vi "Card.vi"(7 "Mode":T1(ring), 8 "error in (no error)":errorcluster, 10 "Queue In":cluster{"Certificate":bool, "Card Info":string}={"Certificate"=TRUE, "Card Info"=""}) -> (0 "error out":errorcluster, 2 "Queue Out":cluster{"Certificate":bool, "Card Info":string}={"Certificate"=TRUE, "Card Info"=""})   [LabVIEW 2011]
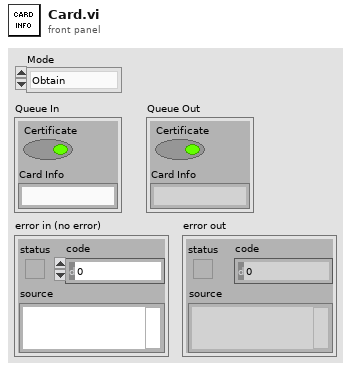
[diagram p1: front panel]
types:
  T1 = enum16{"Obtain", "Enqueue", "Dequeue", "Release"}
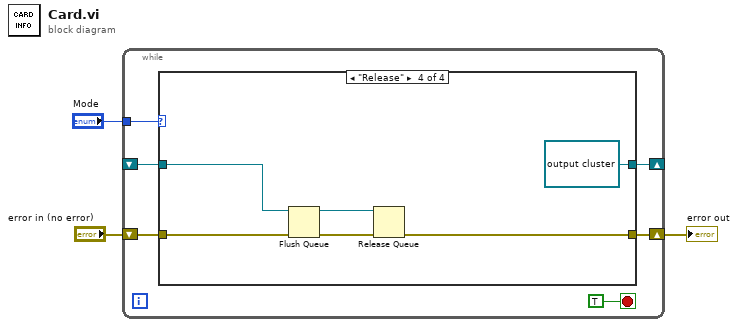
[diagram p0: block diagram]
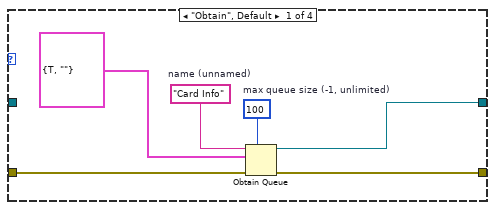
[diagram p2: hidden frame]
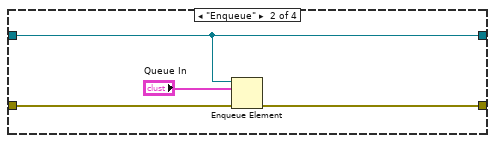
[diagram p3: hidden frame]
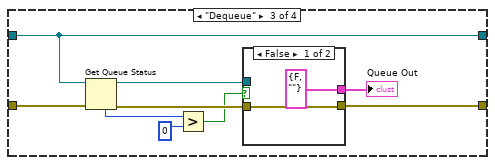
[diagram p4: hidden frame]
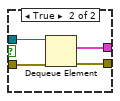
[diagram p5: hidden frame]
diagram:
  n1 = while {
    tunnel: "Mode" -> [w9]
    shift-right: [w7] -> w1
    shift-left: "error in (no error)" -> [w8]
    shift-right: [w6] -> _
    shift-left: _ -> [w5]
    stop <- TRUE stop-if-true
    n2 = case shown="\"Release\"" w9 {
      tunnel: w8 -> [w15 w19 w27 w36]
      tunnel: [w14 w18 w28 w40] -> w7
      tunnel: [w12 w17 w25 refnum<queue> refnum ("queue out")] -> w6
      tunnel: w5 -> [_ w17 w25 w39]
      frame "Obtain", Default {
        w11 = 100  # max queue size (-1, unlimited)
        w13 = "Card Info"  # name (unnamed)
        n3 = Obtain Queue(max queue size (-1, unlimited)=w11, name (unnamed)=w13, element data type=cluster{"Certificate":bool, "Card Info":string} {"Certificate"=TRUE, "Card Info"=""} ("output cluster"), error in (no error)=w15) -> (queue out=w12:refnum<queue>, error out=w14:errorcluster)  [unwired: 1 in, 1 out]
      }
      frame "Enqueue" {
        n4 = Enqueue Element(queue=w17, element="Queue In", error in (no error)=w19) -> (error out=w18:errorcluster)  [unwired: 1 in, 2 out]
      }
      frame "Dequeue" {
        n5 = Get Queue Status(queue=w25, error in (no error)=w27) -> (queue out=w24:refnum<queue>, error out=w26:errorcluster, # elements in queue=w22:i32)  [unwired: 1 in, 5 out]
        n6 = Greater?(x=w22, y=0) -> (0:w21:bool)
        n7 = case shown="False" w21 {
          tunnel: [w30 w34] -> w28
          tunnel: [cluster{"Certificate":bool, "Card Info":string} {"Certificate"=FALSE, "Card Info"=""} ("output cluster") w33] -> w20
          tunnel: w26 -> [w30 w32]
          tunnel: w24 -> [_ w31]
          frame False {
          }
          frame True {
            n8 = Dequeue Element(queue=w31, error in (no error)=w32) -> (element=w33:cluster{"Certificate":bool, "Card Info":string}, error out=w34:errorcluster)  [unwired: 1 in, 2 out]
          }
        }
        "Queue Out" <- w20
      }
      frame "Release" {
        n9 = Flush Queue(queue=w39, error in (no error)=w36) -> (queue out=w37:refnum<queue>, error out=w35:errorcluster)  [unwired: 1 out]
        n10 = Release Queue(queue=w37, error in (no error)=w35) -> (error out=w40:errorcluster)  [unwired: 1 in, 2 out]
      }
    }
  }
  "error out" <- w1
